vi "Decoder.vi"() -> ()   [LabVIEW 2009]
panel:
  in  "stop":bool
  out "3":bool
  out "2":bool
  out "1":bool
  out "0":bool
  in  "Boolean 2":bool
  in  "Boolean":bool
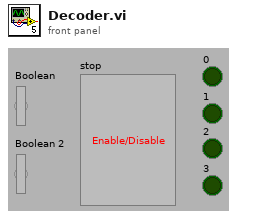
[diagram p1: front panel]
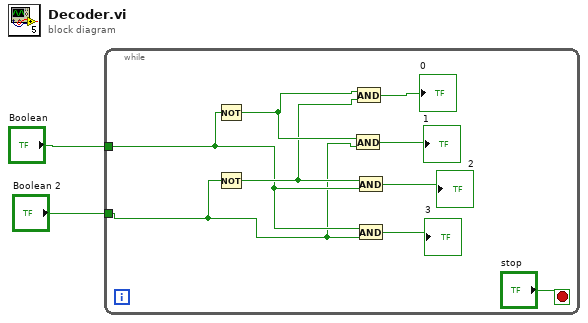
[diagram p0: block diagram]
diagram:
  n1 = while {
    tunnel: "Boolean" -> [w4]
    tunnel: "Boolean 2" -> [w3]
    stop <- "stop" stop-if-true
    n2 = Not(x=w4) -> (.not. x?=w11:bool)
    n3 = Not(x=w3) -> (.not. x?=w10:bool)
    n4 = And(x=w11, y=w3) -> (x .and. y?=→"1":bool)
    n5 = And(x=w11, y=w10) -> (x .and. y?=→"0":bool)
    n6 = And(x=w10, y=w4) -> (x .and. y?=→"2":bool)
    n7 = And(x=w4, y=w3) -> (x .and. y?=→"3":bool)
  }
